vi "load_display_style.vi"(10 "数据显示配置":T1, 11 "Cluster输入":refnum<vi>) -> ()   [LabVIEW 2018, in "UI.lvlib"]
uses:
  UI.lvlib
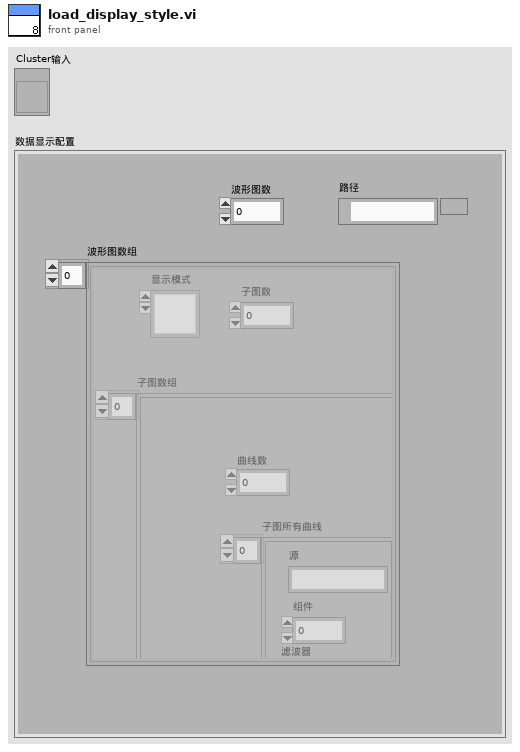
[diagram p1: front panel]
types:
  T1 = typedef "波形图簇.ctl" = cluster{"波形图数":u32, "波形图数组":T2[], "路径":path}
  T2 = typedef "波形图.ctl" = cluster{"显示模式":u16, "子图数":u32, "子图数组":T3[]}
  T3 = typedef "子图.ctl" = cluster{"子图所有曲线":T4[], "曲线数":u32}
  T4 = typedef "曲线簇.ctl" = cluster{"源":string, "组件":u32, "滤波器":u32}
  T5 = enum8{"Enabled", "Disabled", "Disabled and Grayed Out"}
  T6 = typedef "组件常量.ctl" = string[]
  T7 = typedef "滤波器常量.ctl" = string[]
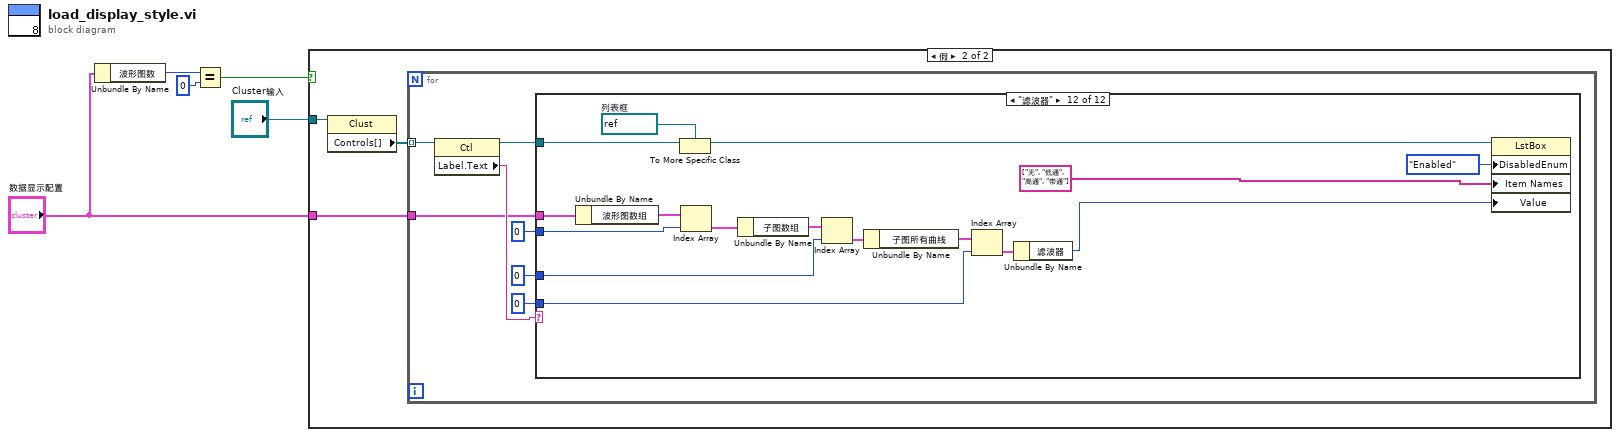
[diagram p0: block diagram]
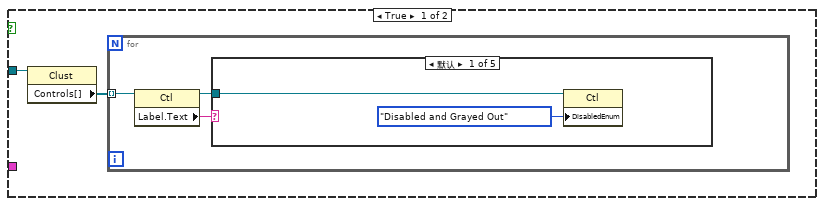
[diagram p2: hidden frame]
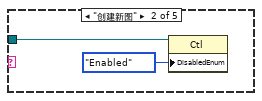
[diagram p3: hidden frame]
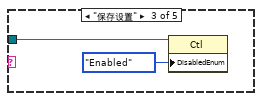
[diagram p4: hidden frame]
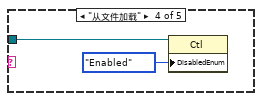
[diagram p5: hidden frame]
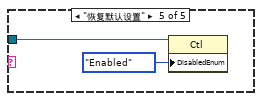
[diagram p6: hidden frame]
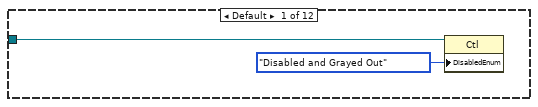
[diagram p7: hidden frame]
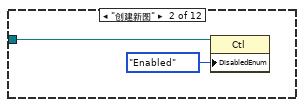
[diagram p8: hidden frame]
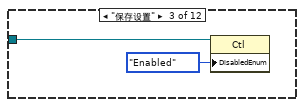
[diagram p9: hidden frame]
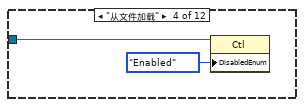
[diagram p10: hidden frame]
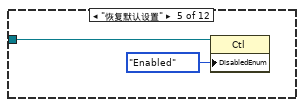
[diagram p11: hidden frame]
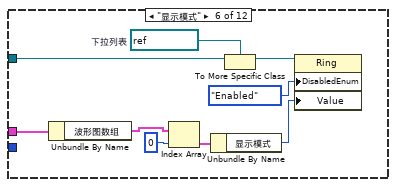
[diagram p12: hidden frame]
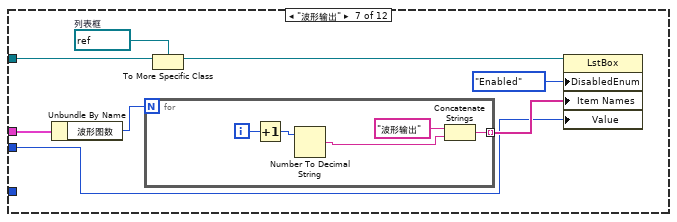
[diagram p13: hidden frame]
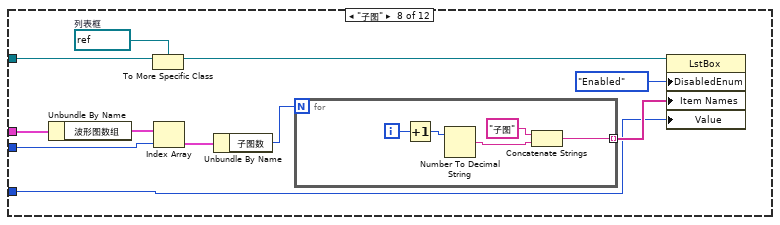
[diagram p14: hidden frame]
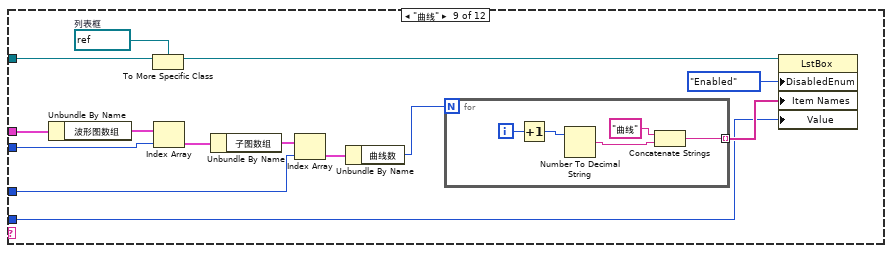
[diagram p15: hidden frame]
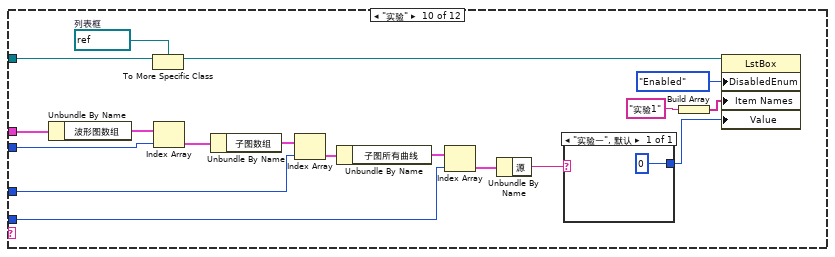
[diagram p16: hidden frame]
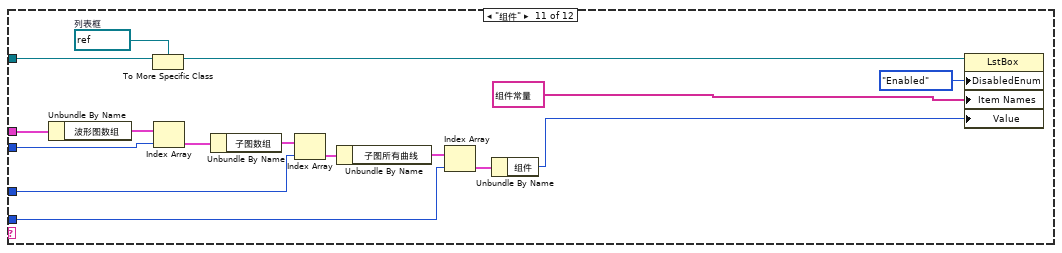
[diagram p17: hidden frame]
diagram:
  n1 = Unbundle By Name("数据显示配置") -> ("波形图数"=w3:u32)
  n2 = Equal?(x=w3, y=0) -> (x = y?=w4:bool)
  n3 = case shown="假" w4 {
    tunnel: "Cluster输入" -> [w7 w23]
    tunnel: "数据显示配置" -> [_ w21]
    frame True {
      n4 = property class="Clust"(reference=w7) -> ("Controls[]"=w6:refnum<vi>[])  [unwired: 1 in, 2 out]
      n5 = for {
        tunnel: w6 -> [w10] mode=indexing
        n6 = property class="Ctl"(reference=w10) -> (reference out=w8:refnum<vi>, "Label.Text"=w9:string)  [unwired: 1 in, 1 out]
        n7 = case shown="默认" w9 {
          tunnel: w8 -> [w12 w14 w16 w18 w20]
          frame Default {
            n8 = property class="Ctl"(reference=w12, "DisabledEnum"=T5."Disabled and Grayed Out" ("禁用")) -> ()  [unwired: 1 in, 2 out]
          }
          frame "创建新图" {
            n9 = property class="Ctl"(reference=w14, "DisabledEnum"=T5."Enabled" ("禁用")) -> ()  [unwired: 1 in, 2 out]
          }
          frame "保存设置" {
            n10 = property class="Ctl"(reference=w16, "DisabledEnum"=T5."Enabled" ("禁用")) -> ()  [unwired: 1 in, 2 out]
          }
          frame "从文件加载" {
            n11 = property class="Ctl"(reference=w18, "DisabledEnum"=T5."Enabled" ("禁用")) -> ()  [unwired: 1 in, 2 out]
          }
          frame "恢复默认设置" {
            n12 = property class="Ctl"(reference=w20, "DisabledEnum"=T5."Enabled" ("禁用")) -> ()  [unwired: 1 in, 2 out]
          }
        }
      }
    }
    frame False {
      n13 = property class="Clust"(reference=w23) -> ("Controls[]"=w22:refnum<vi>[])  [unwired: 1 in, 2 out]
      n14 = for {
        tunnel: w22 -> [w30] mode=indexing
        tunnel: w21 -> [w27]
        n15 = property class="Ctl"(reference=w30) -> (reference out=w28:refnum<vi>, "Label.Text"=w29:string)  [unwired: 1 in, 1 out]
        n16 = case shown="\"滤波器\"" w29 {
          tunnel: w28 -> [w32 w34 w36 w38 w40 w47 w56 w72 w91 w115 w132 w148]
          tunnel: w27 -> [_ _ _ _ _ w48 w53 w69 w88 w112 w129 w145]
          tunnel: 0 -> [_ _ _ _ _ _ _ w66 w81 w107 w124 w140]
          tunnel: 0 -> [_ _ _ _ _ _ w50 w65 w85 w110 w127 w143]
          tunnel: 0 -> [_ _ _ _ _ _ _ _ w82 w104 w121 w137]
          frame Default {
            n17 = property class="Ctl"(reference=w32, "DisabledEnum"=T5."Disabled and Grayed Out" ("禁用")) -> ()  [unwired: 1 in, 2 out]
          }
          frame "创建新图" {
            n18 = property class="Ctl"(reference=w34, "DisabledEnum"=T5."Enabled" ("禁用")) -> ()  [unwired: 1 in, 2 out]
          }
          frame "保存设置" {
            n19 = property class="Ctl"(reference=w36, "DisabledEnum"=T5."Enabled" ("禁用")) -> ()  [unwired: 1 in, 2 out]
          }
          frame "从文件加载" {
            n20 = property class="Ctl"(reference=w38, "DisabledEnum"=T5."Enabled" ("禁用")) -> ()  [unwired: 1 in, 2 out]
          }
          frame "恢复默认设置" {
            n21 = property class="Ctl"(reference=w40, "DisabledEnum"=T5."Enabled" ("禁用")) -> ()  [unwired: 1 in, 2 out]
          }
          frame "显示模式" {
            w45 = refnum<vi> refnum  # 下拉列表
            n22 = Unbundle By Name(w48) -> ("波形图数组"=w44:T2[])
            n23 = Index Array(array=w44, index=0) -> (element=w42:T2)
            n24 = Unbundle By Name(w42) -> ("显示模式"=w41:u16)
            n25 = To More Specific Class(target class=w45, reference=w47) -> (specific class reference=w46:refnum<vi>)  [unwired: 1 in, 1 out]
            n26 = property class="Ring"(reference=w46, "DisabledEnum"=T5."Enabled" ("禁用"), "Value"=w41) -> ()  [unwired: 1 in, 2 out]
          }
          frame "波形输出" {
            w55 = refnum<vi> refnum  # 列表框
            n27 = Unbundle By Name(w53) -> ("波形图数"=w52:u32)
            n28 = for {
              N: w52 -> [_]
              tunnel: [w58] -> w51 mode=indexing
              i -> [w62]
              n29 = Increment(x=w62) -> (x+1=w61:i32)
              n30 = Number To Decimal String(number=w61) -> (decimal integer string=w59:string)  [unwired: 1 in]
              n31 = Concatenate Strings("波形输出", w59) -> (w58:string)
            }
            n32 = To More Specific Class(target class=w55, reference=w56) -> (specific class reference=w54:refnum<vi>)  [unwired: 1 in, 1 out]
            n33 = property class="LstBox"(reference=w54, "DisabledEnum"=T5."Enabled" ("禁用"), "Item Names"=w51, "Value"=w50) -> ()  [unwired: 1 in, 2 out]
          }
          frame "子图" {
            w71 = refnum<vi> refnum  # 列表框
            n34 = Unbundle By Name(w69) -> ("波形图数组"=w67:T2[])
            n35 = To More Specific Class(target class=w71, reference=w72) -> (specific class reference=w70:refnum<vi>)  [unwired: 1 in, 1 out]
            n36 = Index Array(array=w67, index=w65) -> (element=w64:T2)
            n37 = Unbundle By Name(w64) -> ("子图数"=w63:u32)
            n38 = for {
              N: w63 -> [_]
              tunnel: [w74] -> w68 mode=indexing
              i -> [w78]
              n39 = Increment(x=w78) -> (x+1=w77:i32)
              n40 = Number To Decimal String(number=w77) -> (decimal integer string=w75:string)  [unwired: 1 in]
              n41 = Concatenate Strings("子图", w75) -> (w74:string)
            }
            n42 = property class="LstBox"(reference=w70, "DisabledEnum"=T5."Enabled" ("禁用"), "Item Names"=w68, "Value"=w66) -> ()  [unwired: 1 in, 2 out]
          }
          frame "曲线" {
            w90 = refnum<vi> refnum  # 列表框
            n43 = Unbundle By Name(w88) -> ("波形图数组"=w86:T2[])
            n44 = To More Specific Class(target class=w90, reference=w91) -> (specific class reference=w89:refnum<vi>)  [unwired: 1 in, 1 out]
            n45 = Index Array(array=w86, index=w85) -> (element=w84:T2)
            n46 = Unbundle By Name(w84) -> ("子图数组"=w83:T3[])
            n47 = Index Array(array=w83, index=w81) -> (element=w80:T3)
            n48 = Unbundle By Name(w80) -> ("曲线数"=w79:u32)
            n49 = for {
              N: w79 -> [_]
              tunnel: [w93] -> w87 mode=indexing
              i -> [w97]
              n50 = Increment(x=w97) -> (x+1=w96:i32)
              n51 = Number To Decimal String(number=w96) -> (decimal integer string=w94:string)  [unwired: 1 in]
              n52 = Concatenate Strings("曲线", w94) -> (w93:string)
            }
            n53 = property class="LstBox"(reference=w89, "DisabledEnum"=T5."Enabled" ("禁用"), "Item Names"=w87, "Value"=w82) -> ()  [unwired: 1 in, 2 out]
          }
          frame "实验" {
            w114 = refnum<vi> refnum  # 列表框
            n54 = Unbundle By Name(w112) -> ("波形图数组"=w111:T2[])
            n55 = To More Specific Class(target class=w114, reference=w115) -> (specific class reference=w113:refnum<vi>)  [unwired: 1 in, 1 out]
            n56 = Index Array(array=w111, index=w110) -> (element=w109:T2)
            n57 = Unbundle By Name(w109) -> ("子图数组"=w108:T3[])
            n58 = Index Array(array=w108, index=w107) -> (element=w106:T3)
            n59 = Unbundle By Name(w106) -> ("子图所有曲线"=w105:T4[])
            n60 = Index Array(array=w105, index=w104) -> (element=w103:T4)
            n61 = Unbundle By Name(w103) -> ("源"=w99:string)
            n62 = case shown="\"实验一\", 默认" w99 {
              tunnel: [0] -> w98
              frame "实验一", Default {
              }
            }
            n63 = Build Array("实验1") -> (w100:string[])
            n64 = property class="LstBox"(reference=w113, "DisabledEnum"=T5."Enabled" ("禁用"), "Item Names"=w100, "Value"=w98) -> ()  [unwired: 1 in, 2 out]
          }
          frame "组件" {
            w131 = refnum<vi> refnum  # 列表框
            n65 = Unbundle By Name(w129) -> ("波形图数组"=w128:T2[])
            n66 = To More Specific Class(target class=w131, reference=w132) -> (specific class reference=w130:refnum<vi>)  [unwired: 1 in, 1 out]
            n67 = Index Array(array=w128, index=w127) -> (element=w126:T2)
            n68 = Unbundle By Name(w126) -> ("子图数组"=w125:T3[])
            n69 = Index Array(array=w125, index=w124) -> (element=w123:T3)
            n70 = Unbundle By Name(w123) -> ("子图所有曲线"=w122:T4[])
            n71 = Index Array(array=w122, index=w121) -> (element=w120:T4)
            n72 = Unbundle By Name(w120) -> ("组件"=w117:u32)
            n73 = property class="LstBox"(reference=w130, "DisabledEnum"=T5."Enabled" ("禁用"), "Item Names"=T6 ["正弦", "方波", "三角", "锯齿"] ("数组"), "Value"=w117) -> ()  [unwired: 1 in, 2 out]
          }
          frame "滤波器" {
            w147 = refnum<vi> refnum  # 列表框
            n74 = Unbundle By Name(w145) -> ("波形图数组"=w144:T2[])
            n75 = To More Specific Class(target class=w147, reference=w148) -> (specific class reference=w146:refnum<vi>)  [unwired: 1 in, 1 out]
            n76 = Index Array(array=w144, index=w143) -> (element=w142:T2)
            n77 = Unbundle By Name(w142) -> ("子图数组"=w141:T3[])
            n78 = Index Array(array=w141, index=w140) -> (element=w139:T3)
            n79 = Unbundle By Name(w139) -> ("子图所有曲线"=w138:T4[])
            n80 = Index Array(array=w138, index=w137) -> (element=w136:T4)
            n81 = Unbundle By Name(w136) -> ("滤波器"=w133:u32)
            n82 = property class="LstBox"(reference=w146, "DisabledEnum"=T5."Enabled" ("禁用"), "Item Names"=T7 ["无", "低通", "高通", "带通"] ("数组"), "Value"=w133) -> ()  [unwired: 1 in, 2 out]
          }
        }
      }
    }
  }
